vi "sensor_de_toque.vi"(1 "valor_eixo":dbl) -> (8 "parada":dbl)   [LabVIEW 2020]
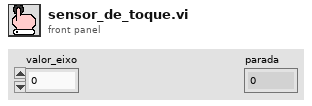
[diagram p1: front panel]
types:
  T1 = typedef "WPI_DigitalInputDevRef.ctl" = cluster{"DevStatus":errorcluster, "DIO Channel":T2}
  T2 = typedef "FPGA_DIOChannel.ctl" = enum8{"DIO 0", "DIO 1", "DIO 2", "DIO 3", "DIO 4", "DIO 5", "DIO 6", "DIO 7", "DIO 8", "DIO 9", "DIO MXP 0", "DIO MXP 1", "DIO MXP 2", "DIO MXP 3", "DIO MXP 4", "DIO MXP 5", "DIO MXP 6", "DIO MXP 7", "DIO MXP 8", "DIO MXP 9", "DIO MXP 10", "DIO MXP 11", "DIO MXP 12", "DIO MXP 13", "DIO MXP 14", "DIO MXP 15", "SPI Port CS1", "SPI Port CS2", "SPI Port CS3", "SPI Port MISO", "SPI Port MOSI", "Invalid"}
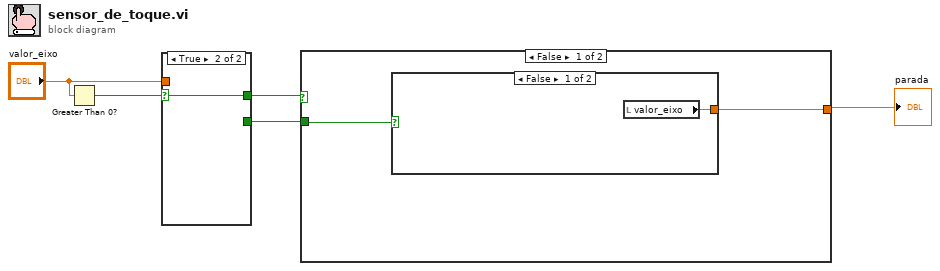
[diagram p0: block diagram]
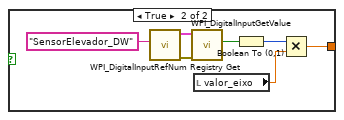
[diagram p2: hidden frame]
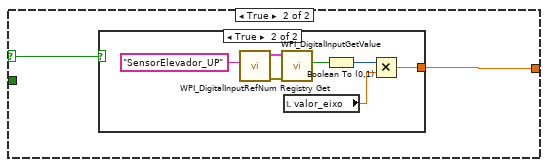
[diagram p3: hidden frame]
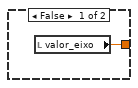
[diagram p4: hidden frame]
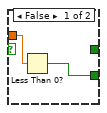
[diagram p5: hidden frame]
diagram:
  n1 = Greater Than 0?(x="valor_eixo") -> (x > 0?=w5:bool)
  n2 = case shown="True" w5 {
    selector: w5 -> [_ w8]
    tunnel: [w6 _] -> w2
    tunnel: [_ w8] -> w1
    tunnel: "valor_eixo" -> [w7 _]
    frame False {
      n3 = Less Than 0?(x=w7) -> (x < 0?=w6:bool)
    }
    frame True {
    }
  }
  n4 = case shown="False" w1 {
    selector: w1 -> [_ w19]
    tunnel: [w10 w20] -> w3
    tunnel: w2 -> [w9 _]
    frame False {
      n5 = case shown="False" w9 {
        tunnel: [w11 w14] -> w10
        frame False {
          n6 = local read "valor_eixo"() -> (w11:dbl)
        }
        frame True {
          n7 = call <vilib>:"WPI_DigitalInputRefNum Registry Get.vi"("refnum name"="SensorElevador_DW") -> ("error out"=w17:errorcluster, "DigitalInputDevRef"=w18:T1)  [unwired: 9 in]
          n8 = call <vilib>:"WPI_DigitalInputGetValue.vi"("error in (no error)"=w17, "DigitalInputDevRef"=w18) -> ("Value"=w13:bool)  [unwired: 7 in, 2 out]
          n9 = local read "valor_eixo"() -> (w15:dbl)
          n10 = Boolean To (0,1)(Boolean=w13) -> (0, 1=w12:i16)
          n11 = Multiply(x=w12, y=w15) -> (x*y=w14:dbl)
        }
      }
    }
    frame True {
      n12 = case shown="True" w19 {
        tunnel: [w21 w24] -> w20
        frame False {
          n13 = local read "valor_eixo"() -> (w21:dbl)
        }
        frame True {
          n14 = call <vilib>:"WPI_DigitalInputRefNum Registry Get.vi"("refnum name"="SensorElevador_UP") -> ("error out"=w28:errorcluster, "DigitalInputDevRef"=w27:T1)  [unwired: 9 in]
          n15 = call <vilib>:"WPI_DigitalInputGetValue.vi"("error in (no error)"=w28, "DigitalInputDevRef"=w27) -> ("Value"=w22:bool)  [unwired: 7 in, 2 out]
          n16 = local read "valor_eixo"() -> (w25:dbl)
          n17 = Boolean To (0,1)(Boolean=w22) -> (0, 1=w23:i16)
          n18 = Multiply(x=w23, y=w25) -> (x*y=w24:dbl)
        }
      }
    }
  }
  "parada" <- w3
